vi "Find Label.vi"(8 "error in":errorcluster, 9 "SDI value":T2=-1 items=["All"=-1, "0 (b00)"=0, "1 (b01)"=1, "2 (b10)"=2, "3 (b11)"=3], 10 "label value":u32, 11 "port in":T1 format="%.0x") -> (0 "error out":errorcluster, 2 "label":T1 format="%.0x", 3 "port out":T1 format="%.0x", 4 "found?":bool)   [LabVIEW 2020, in "Ballard ARINC 429 Scripting.lvlib"]
doc: "Under the specified port, searches for a label with matching <b>label value</b> and <b>SDI value</b>. If a match is found, returns the matching <b>label</b> reference. If no match is found, the returned reference is invalid and <b>found?</b> equals False."
uses:
  Ballard ARINC 429 Scripting.lvlib
  Shared/SDI.ctl
  <vilib>/NI VeriStand/Custom Device API/Custom Device Item Ref.ctl
  Shared/Label Properties.ctl
  Shared/Label.ctl
  <vilib>/NI VeriStand/Custom Device API/Custom Device API.lvlib
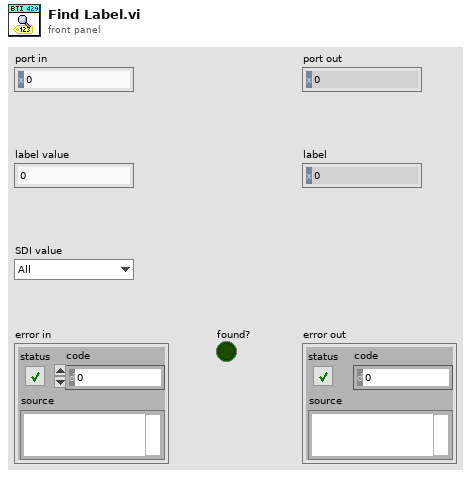
[diagram p1: front panel]
types:
  T1 = typedef "Custom Device API.lvlib/Custom Device Item Ref.ctl" = u64
  T2 = typedef "SDI.ctl" = i32
  T3 = typedef "Label Properties.ctl" = cluster{"label (Dec)":T4, "SDI value":u8, "SDI enabled":bool}
  T4 = typedef "Label.ctl" = u8
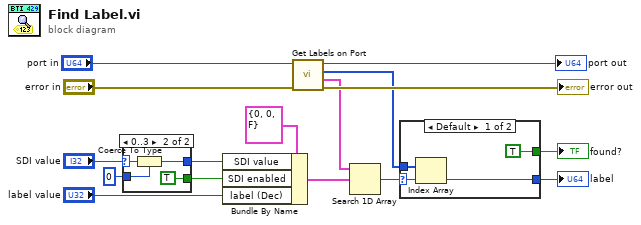
[diagram p0: block diagram]
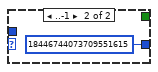
[diagram p2: hidden frame]
diagram:
  n1 = case shown="0..3" "SDI value" {
    selector: "SDI value" -> [_ w20]
    tunnel: [w17 w21] -> w8
    tunnel: u8 0 ("SDI value") -> [w17 w19]
    tunnel: [_ TRUE] -> w7
    frame Default {
    }
    frame 0..3 {
      n2 = Coerce To Type(0:w20, 1:w19) -> (2:w21:u8)
    }
  }
  n3 = Bundle By Name(cluster=T3 {"label (Dec)"=0, "SDI value"=0, "SDI enabled"=FALSE} ("label properties"), "SDI value"=w8, "SDI enabled"=w7, "label (Dec)"="label value") -> (w5:T3)
  n4 = call "Get Labels on Port.vi"("error in"="error in", "port in"="port in") -> ("error out"=→"error out":errorcluster, "labels properties"=w6:T3[], "labels"=w3:T1[], "port out"=→"port out":T1)  [unwired: 6 in]
  n5 = Search 1D Array(1D array=w6, element=w5) -> (index of element=w4:i32)  [unwired: 1 in]
  n6 = case shown="Default" w4 {
    selector: w4 -> [w24 _]
    tunnel: w3 -> [w25 _]
    tunnel: [w23 T1 18446744073709551615 ("Invalid Ref")] -> w1
    tunnel: [TRUE _] -> w2
    frame Default {
      n7 = Index Array(array=w25, index=w24) -> (element=w23:T1)
    }
    frame ..-1 {
    }
  }
  "label" <- w1
  "found?" <- w2
